vi "ReadGUID.vi"() -> (3 "Array":string[](array[string]))   [LabVIEW 2017]
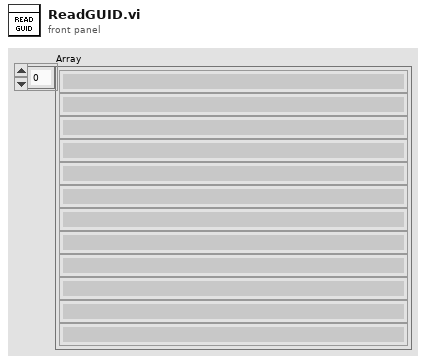
[diagram p1: front panel]
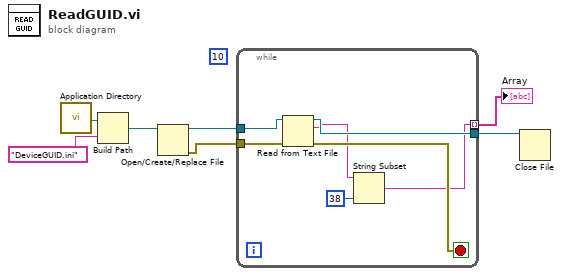
[diagram p0: block diagram]
diagram:
  (unwired) 10
  n1 = call <vilib>:"Application Directory.vi"() -> ("Application Directory"=w7:path)
  n2 = Build Path(base path=w7, name or relative path="DeviceGUID.ini") -> (appended path=w5:path)
  n3 = Open/Create/Replace File(file path (use dialog)=w5) -> (refnum out=w4:refnum<file>, error out=w1:errorcluster)  [unwired: 5 in, 1 out]
  n4 = while {
    tunnel: w4 -> [w14]
    tunnel: [w13] -> w3
    tunnel: [w8] -> w2 mode=indexing
    tunnel: w1 -> [w11]
    stop <- w12 stop-if-true
    n5 = Read from Text File(file (use dialog)=w14, error in=w11) -> (refnum out=w13:refnum<file>, text=w10:string, error out=w12:errorcluster)  [unwired: 2 in, 1 out]
    n6 = String Subset(string=w10, length (rest)=38 ("length (rest)")) -> (substring=w8:string)  [unwired: 1 in]
  }
  "Array" <- w2
  n7 = Close File(refnum=w3) -> ()  [unwired: 1 in, 2 out]
